vi "Set LibraryPaths to Include Icon Editor.vi"(8 "error in (no error)":errorcluster) -> (0 "error out":errorcluster, 3 "config modified?":bool)   [LabVIEW 2020]
uses:
  <vilib>/Utility/config.llb/NI_LVConfig.lvlib
  <vilib>/Utility/config.llb/Read Key (String).vi
  <vilib>/Utility/config.llb/Write Key (String).vi
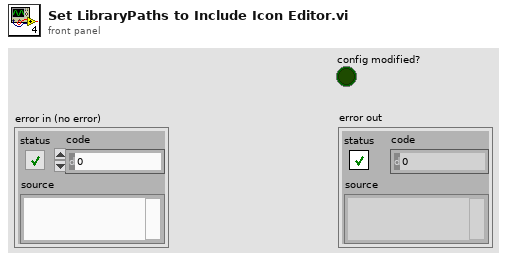
[diagram p1: front panel]
types:
  T1 = typedef "NI_LVConfig.lvlib/Config Data RefNum.ctl" = refnum<k1>
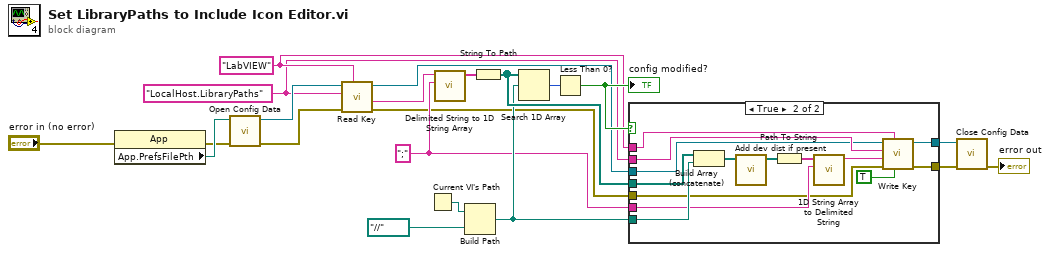
[diagram p0: block diagram]
diagram:
  w11 = ";" ("delimiter")
  w10 = "LabVIEW" ("section")
  w9 = "LocalHost.LibraryPaths" ("key")
  n1 = property class="App"(error in="error in (no error)") -> (error out=w6:errorcluster, "App.PrefsFilePth"=w21:path)  [unwired: 1 in, 1 out]
  n2 = call <vilib>:"Open Config Data.vi"("error in (no error)"=w6, "configuration file path"=w21) -> ("error out"=w7:errorcluster, "refnum"=w20:T1)  [unwired: 7 in, 1 out]
  n3 = call-poly <vilib>:"Read Key.vi"("section"=w10, "error in (no error)"=w7, "key"=w9, "refnum"=w20) -> ("error out"=w5:errorcluster, "value"=w17:string, "refnum out"=w8:T1)  [unwired: 4 in, 1 out]
  n4 = Current VI's Path() -> (path=w18:path)
  n5 = call <vilib>:"Delimited String to 1D String Array.vi"("delimiter"=w11, "delimited string"=w17) -> ("string array"=w16:string[])  [unwired: 9 in]
  n6 = Build Path(base path=w18, name or relative path=path "../../..") -> (appended path=w12:path)
  n7 = String To Path(string=w16) -> (path=w13:path[])
  n8 = Search 1D Array(1D array=w13, element=w12) -> (index of element=w15:i32)  [unwired: 1 in]
  n9 = Less Than 0?(x=w15) -> (x < 0?=w14:bool)
  "config modified?" <- w14
  n10 = case shown="True" w14 {
    tunnel: w13 -> [_ w37]
    tunnel: w12 -> [_ w36]
    tunnel: w11 -> [_ w33]
    tunnel: w10 -> [_ w32]
    tunnel: w9 -> [_ w31]
    tunnel: w8 -> [w23 w29]
    tunnel: w5 -> [w22 w28]
    tunnel: [w23 w27] -> w4
    tunnel: [w22 w26] -> w3
    frame False {
    }
    frame True {
      n11 = Build Array (concatenate)(w37, w36) -> (w35:path[])
      n12 = call "Add dev dist if present.vi"("paths in"=w35) -> ("paths out"=w24:path[])  [unwired: 10 in]
      n13 = Path To String(path=w24) -> (string=w34:string[])
      n14 = call <vilib>:"1D String Array to Delimited String.vi"("delimiter"=w33, "string array"=w34) -> ("delimited string"=w30:string)  [unwired: 9 in]
      n15 = call-poly <vilib>:"Write Key.vi"("write raw string? (F)"=TRUE, "section"=w32, "error in (no error)"=w28, "value"=w30, "key"=w31, "refnum"=w29) -> ("error out"=w26:errorcluster, "refnum out"=w27:T1)  [unwired: 3 in, 1 out]
    }
  }
  n16 = call <vilib>:"Close Config Data.vi"("error in (no error)"=w3, "refnum"=w4) -> ("error out"=→"error out":errorcluster)  [unwired: 8 in, 1 out]
